vi "Deadzone.vi"(2 "Deadzone":dbl, 3 "Input Signal":dbl) -> (0 "Output Signal":dbl, 1 "In Deadzone":bool)   [LabVIEW 2013]
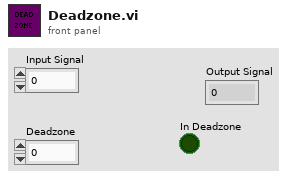
[diagram p1: front panel]
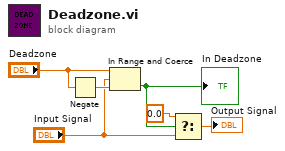
[diagram p0: block diagram]
diagram:
  n1 = Negate(x="Deadzone") -> (-x=w5:dbl)
  n2 = In Range and Coerce(upper limit="Deadzone", x="Input Signal", lower limit=w5) -> (In Range?=w4:bool)  [unwired: 1 out]
  "In Deadzone" <- w4
  n3 = Select(t=0.0, s=w4, f="Input Signal") -> (s? t:f=→"Output Signal":dbl)
